vi "G#Object_RegisterObject.vi"(0 "reference in":refnum<class "G#Object.lvclass">, 1 "attribute refs":u32[](array[numeric]), 3 "created new":bool, 4 "no registration":bool, 5 "error in (no error)":errorcluster) -> (14 "reference out":refnum<class "G#Object.lvclass">, 19 "error out":errorcluster)   [LabVIEW 2020, in "G#Object.lvclass"]
doc: "Registers the object to the G# all objects lists. It also sends an event to the debugger and the desktop trace."
uses:
  G#Object.lvclass
  G#Object.lvclass/G#Object.ctl
  utils/G#Object_EventType.ctl
  utils/G#Object_ObjectInfoType.ctl
  utils/G#Object_CreateMethod.ctl
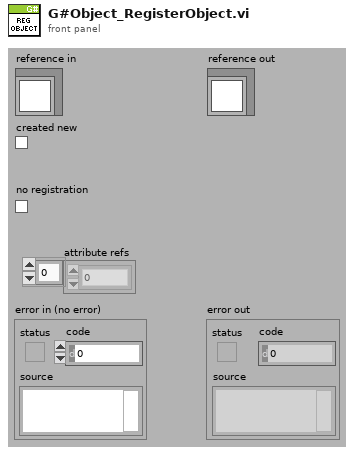
[diagram p1: front panel]
types:
  T1 = typedef "G#Object.lvclass/G#Object_EventType.ctl" = enum16{"Created new", "Looked up existing", "Deleted", "Forced delete", "Not deleted", "Garbage collected", "Cleared", "User", "Error", "External create object", "External create class attributes", "Created class attributes", "Run constructor", "Run constructor done", "Run open method", "Run open method done"}
  T2 = typedef "G#Object.lvclass/G#Object_ObjectInfoType.ctl" = cluster{"ObjectName":string, "ObjectID":u32, "Users":i32, "Counter":bool, "AttributeRefs":u32[], "FullClassName":string, "ClassName":string, "CreateMethod":T3, "GenericDestructorExists":bool, "Owner":string}
  T3 = typedef "G#Object.lvclass/G#Object_CreateMethod.ctl" = enum16{"Create", "Create or look up existing", "Look up existing"}
  T4 = cluster{"FullClassName":string, "reference in":refnum<class "G#Object.lvclass">}
  T5 = cluster{"FullClassName":string, "reference in":refnum<class "G#Object.lvclass">}[]
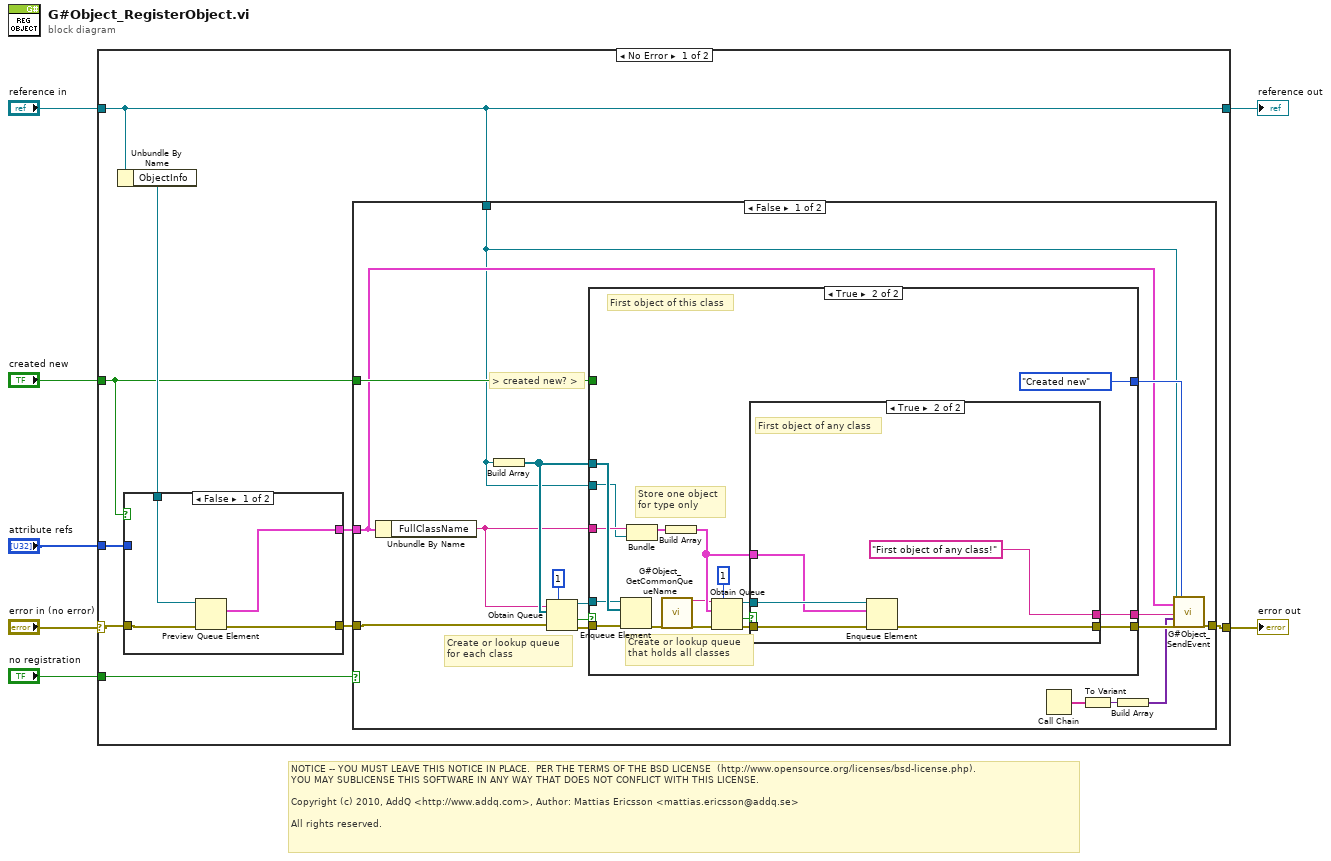
[diagram p0: block diagram]
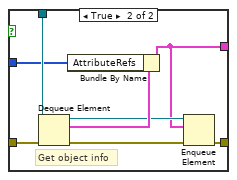
[diagram p2: hidden frame]
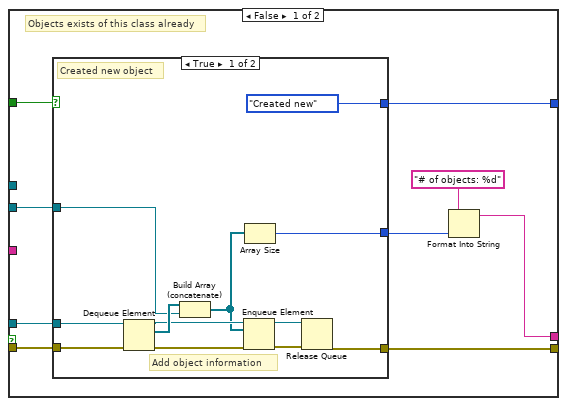
[diagram p3: hidden frame]
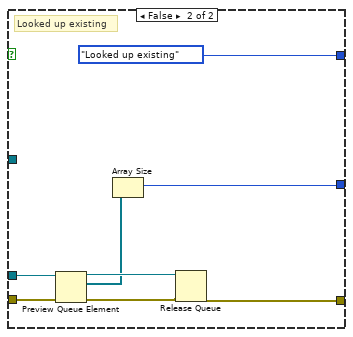
[diagram p4: hidden frame]
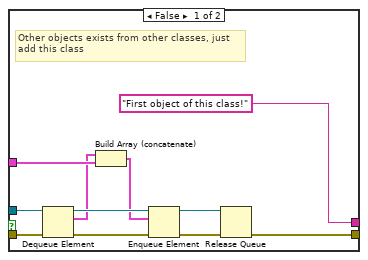
[diagram p5: hidden frame]
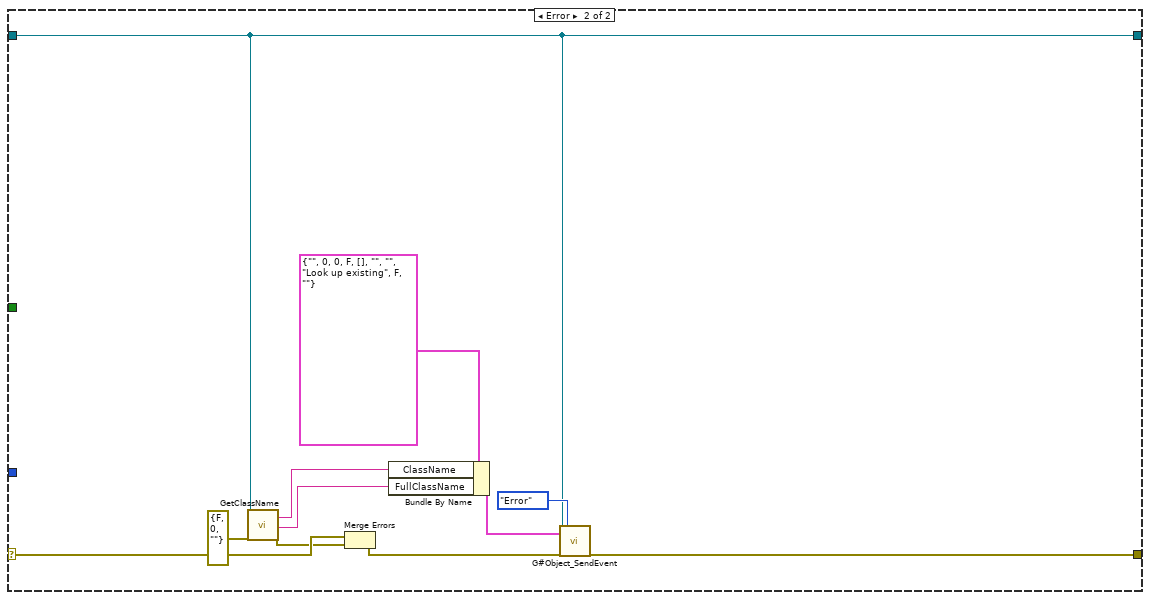
[diagram p7: hidden frame]
diagram:
  # "NOTICE -- YOU MUST LEAVE THIS NOTICE IN PLACE.  PER THE TERMS OF THE BSD LICENSE  (http://www.opensource.org/licenses/bsd-license.php).\nYOU MAY SUBLICENSE THIS SOFTWARE IN ANY WAY THAT DOES NOT CONFLICT WITH THIS LICENSE.\n\nCopyright (c) 2010, AddQ <http://www.addq.com>, Author: Mattias Ericsson <mattias.ericsson@addq.se>\n\nAll rights reserved."
  n1 = case shown="No Error" "error in (no error)" {
    selector: "error in (no error)" -> [w15 w117]
    tunnel: [w16 w119] -> w6
    tunnel: [w11 w113] -> w4
    tunnel: "reference in" -> [w11 w113]
    tunnel: "created new" -> [w8 _]
    tunnel: "no registration" -> [w10 _]
    tunnel: "attribute refs" -> [w9 _]
    frame No Error {
      n2 = Unbundle By Name(w11) -> ("ObjectInfo"=w13:refnum<queue>)
      n3 = case shown="False" w8 {
        tunnel: w15 -> [w20 w26]
        tunnel: [w18 w24] -> w14
        tunnel: w13 -> [w19 w23]
        tunnel: [w17 w22] -> w12
        tunnel: w9 -> [_ w21]
        frame False {
          n4 = Preview Queue Element(queue=w19, error in (no error)=w20) -> (element=w17:T2, error out=w18:errorcluster)  [unwired: 1 in, 2 out]
        }
        frame True {
          # "Get object info"
          n5 = Dequeue Element(queue=w23, error in (no error)=w26) -> (queue out=w27:refnum<queue>, element=w28:T2, error out=w25:errorcluster)  [unwired: 1 in, 1 out]
          n6 = Bundle By Name(cluster=w28, "AttributeRefs"=w21) -> (w22:T2)
          n7 = Enqueue Element(queue=w27, element=w22, error in (no error)=w25) -> (error out=w24:errorcluster)  [unwired: 1 in, 2 out]
        }
      }
      n8 = case shown="False" w10 {
        tunnel: w8 -> [w37 _]
        tunnel: [w35 w108] -> w16
        tunnel: w14 -> [w29 w108]
        tunnel: w12 -> [w34 _]
        tunnel: w11 -> [w33 _]
        frame False {
          # "> created new? >"
          # "Create or lookup queue\nfor each class"
          n9 = Unbundle By Name(w34) -> ("FullClassName"=w36:string)
          n10 = Build Array(w33) -> (w41:refnum<class "G#Object.lvclass">[])
          n11 = Obtain Queue(max queue size (-1, unlimited)=1, name (unnamed)=w36, element data type=w41, error in (no error)=w29) -> (queue out=w42:refnum<queue>, created new?=w43:bool, error out=w44:errorcluster)  [unwired: 1 in]
          n12 = case shown="True" w43 {
            tunnel: w44 -> [w54 w89]
            tunnel: w42 -> [w53 w90]
            tunnel: w41 -> [_ w91]
            tunnel: [w52 w88] -> w40
            tunnel: w36 -> [_ w80]
            tunnel: w37 -> [w51 _]
            tunnel: [w50 G#Object_EventType."Created new" ("G#Event")] -> w39
            tunnel: [w46 w81] -> w38
            tunnel: w33 -> [w49 w78]
            frame False {
              # "Objects exists of this class already"
              n13 = case shown="True" w51 {
                tunnel: w54 -> [w66 w71]
                tunnel: w53 -> [w65 w72]
                tunnel: [w61 w74] -> w52
                tunnel: [G#Object_EventType."Created new" ("G#Event") G#Object_EventType."Looked up existing" ("G#Event")] -> w50
                tunnel: w49 -> [w57 _]
                tunnel: [w55 w67] -> w47
                frame True {
                  # "Created new object"
                  # "Add object information"
                  n14 = Dequeue Element(queue=w65, error in (no error)=w66) -> (queue out=w63:refnum<queue>, element=w64:refnum<class "G#Object.lvclass">[], error out=w62:errorcluster)  [unwired: 1 in, 1 out]
                  n15 = Build Array (concatenate)(w64, w57) -> (w56:refnum<class "G#Object.lvclass">[])
                  n16 = Enqueue Element(queue=w63, element=w56, error in (no error)=w62) -> (queue out=w59:refnum<queue>, error out=w60:errorcluster)  [unwired: 1 in, 1 out]
                  n17 = Array Size(array=w56) -> (size(s)=w55:i32)
                  n18 = Release Queue(queue=w59, error in (no error)=w60) -> (error out=w61:errorcluster)  [unwired: 1 in, 2 out]
                }
                frame False {
                  # "Looked up existing"
                  n19 = Preview Queue Element(queue=w72, error in (no error)=w71) -> (queue out=w69:refnum<queue>, element=w68:refnum<class "G#Object.lvclass">[], error out=w70:errorcluster)  [unwired: 1 in, 1 out]
                  n20 = Array Size(array=w68) -> (size(s)=w67:i32)
                  n21 = Release Queue(queue=w69, error in (no error)=w70) -> (error out=w74:errorcluster)  [unwired: 1 in, 2 out]
                }
              }
              n22 = Format Into String(format string="# of objects: %d", w47) -> (resulting string=w46:string)  [unwired: 2 in, 1 out]
            }
            frame True {
              # "Store one object\nfor type only"
              # "Create or lookup queue\nthat holds all classes"
              # "First object of this class"
              n23 = Enqueue Element(queue=w90, element=w91, error in (no error)=w89) -> (error out=w77:errorcluster)  [unwired: 1 in, 2 out]
              n24 = Bundle("FullClassName"=w80, "reference in"=w78) -> (w79:T4)  [unwired: 1 in]
              n25 = call "G#Object_GetCommonQueueName.vi"("error in (no error)"=w77) -> ("queue name"=w75:string, "error out"=w76:errorcluster)  [unwired: 17 in]
              n26 = Build Array(w79) -> (w84:T5)
              n27 = Obtain Queue(max queue size (-1, unlimited)=1, name (unnamed)=w75, element data type=w84, error in (no error)=w76) -> (queue out=w86:refnum<queue>, created new?=w85:bool, error out=w87:errorcluster)  [unwired: 1 in]
              n28 = case shown="True" w85 {
                tunnel: w87 -> [w102 w107]
                tunnel: [w96 w106] -> w88
                tunnel: w86 -> [w101 w105]
                tunnel: w84 -> [w94 w104]
                tunnel: ["First object of this class!" "First object of any class!"] -> w81
                frame False {
                  # "Other objects exists from other classes, just\nadd this class"
                  n29 = Dequeue Element(queue=w101, error in (no error)=w102) -> (queue out=w100:refnum<queue>, element=w93:T5, error out=w97:errorcluster)  [unwired: 1 in, 1 out]
                  n30 = Build Array (concatenate)(w93, w94) -> (w95:T5)
                  n31 = Enqueue Element(queue=w100, element=w95, error in (no error)=w97) -> (queue out=w98:refnum<queue>, error out=w99:errorcluster)  [unwired: 1 in, 1 out]
                  n32 = Release Queue(queue=w98, error in (no error)=w99) -> (error out=w96:errorcluster)  [unwired: 1 in, 2 out]
                }
                frame True {
                  # "First object of any class"
                  n33 = Enqueue Element(queue=w105, element=w104, error in (no error)=w107) -> (error out=w106:errorcluster)  [unwired: 1 in, 2 out]
                }
              }
            }
          }
          n34 = Call Chain() -> (call chain=w30:string[])
          n35 = To Variant(anything=w30) -> (Variant=w32:variant)
          n36 = Build Array(w32) -> (w31:variant[])
          n37 = call "G#Object_SendEvent.vi"("reference in"=w33, "object info extended"=w34, "comment"=w38, "parameters"=w31, "error in (no error)"=w40, "G# event type"=w39) -> ("error out"=w35:errorcluster)  [unwired: 13 in]
        }
        frame True {
        }
      }
    }
    frame Error {
      n38 = call-dynamic "GetClassName.vi"("reference in"=w113, "error in (no error)"=errorcluster {"status"=FALSE, "code"=0, "source"=""}) -> ("class name"=w110:string, "full class name"=w109:string, "error out"=w116:errorcluster)  [unwired: 13 in, 2 out]
      n39 = Merge Errors(w117, w116) -> (w114:errorcluster)
      n40 = Bundle By Name(cluster=T2 {"ObjectName"="", "ObjectID"=0, "Users"=0, "Counter"=FALSE, "AttributeRefs"=[], "FullClassName"="", "ClassName"="", "CreateMethod"=enum."Look up existing", "GenericDestructorExists"=FALSE, "Owner"=""}, "ClassName"=w110, "FullClassName"=w109) -> (w111:T2)
      n41 = call "G#Object_SendEvent.vi"("reference in"=w113, "object info extended"=w111, "error in (no error)"=w114, "G# event type"=G#Object_EventType."Error") -> ("error out"=w119:errorcluster)  [unwired: 15 in]
    }
  }
  "error out" <- w6
  "reference out" <- w4
